vi "MCP3208 SPI Analog Input.vi"   [LabVIEW 2014]
doc: "This example shows how to read ADC value from MCP3208."
uses:
  QwaveSys_Interface/QwaveSys_Interface.lvlib
  PWS_ESP8266/PWS_ESP8266.lvlib
panel:
  # "Overview: Demonstrates how to read ADC data from MCP3208, Refer at this link: http://ww1.microchip.com/downloads/en/DeviceDoc/21298c.pdf\nRequirements: LabVIEW Full Development System,Arduino Compatible Compiler for LabVIEW,Programmable Wireless Stamp (PWS) Library.\nInstructions:\n1. Wire the MCP3208 IC to the Pmod SPI interface. refer below diagram.\n2. If this example has been loaded from the Arduino Compatible Compiler for LabVIEW, simply select Compile and Download.  Otherwise, open Tools>Arduino Compatible Compiler for LabVIEW in LabVIEW, then select File>Load VI, and select this VI and then Compile and Download.\n3. Open \"Serial Monitor\" by select \"Tools>Serial Monitor\" and select baud rate to 9600.\n4. Observe the data \"ADC 8 ch single end & 4 ch differential\" being print out on serial port monitor.\n\n#NOTE: \nThe MCP3208 chip is a very popular successive approximation 12-Bit ADC with SPI interface. The chip is programmable to provide four pseudo-differential input pairs or eight single-ended inputs and is capable of sample rates up to 100 Ksps. Custom designs or off the shelf modules utilizing the MCP3208 is a great option in case the user needs ADC channels with higher resolution than the 10-bit ADC that is included as part of the PWS.\nrefer: http://ww1.microchip.com/downloads/en/DeviceDoc/21298c.pdf"
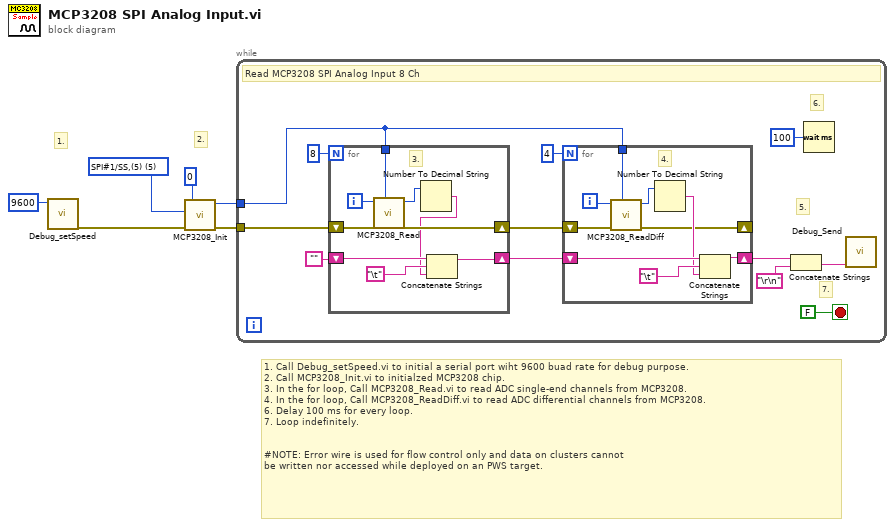
[diagram p0: block diagram]
diagram:
  w1 = u8 5 items=["SPI#1/SS,(5)"=5, "SPI#2/MOSI,(13)"=13, "SPI#3/MISO,(12)"=12, "SPI#4/SCLK,(14)"=14, "UART#1/CS,(15)"=15, "UART#2/TXD,(1)"=1, "UART#3/RXD,(3)"=3, "UART#4/LED,(16)"=16, "FPROM_Btn,(0)"=0, "SDCard_CS,(4)"=4, "I2C-SDA/TXD1,(2)"=2, "ADC0,(17)"=17] ("CS")
  # "2."
  # "1."
  # "1. Call Debug_setSpeed.vi to initial a serial port wiht 9600 buad rate for debug purpose.\n2. Call MCP3208_Init.vi to initialzed MCP3208 chip.\n3. In the for loop, Call MCP3208_Read.vi to read ADC single-end channels from MCP3208.\n4. In the for loop, Call MCP3208_ReadDiff.vi to read ADC differential channels from MCP3208.\n6. Delay 100 ms for every loop.\n7. Loop indefinitely.\n\n\n#NOTE: Error wire is used for flow control only and data on clusters cannot\nbe written nor accessed while deployed on an PWS target."
  n1 = call "Debug_setSpeed.vi"("Speed"=u32 9600) -> ("error out"=w3:errorcluster)  [unwired: 10 in]
  n2 = call "MCP3208_Init.vi"("error in"=w3, "CS"=w1, "Interface (0-4)"=u8 0) -> ("error out"=w4:errorcluster, "Instance"=w5:u8)  [unwired: 7 in]
  n3 = while {
    tunnel: w5 -> [w13]
    tunnel: w4 -> [w18]
    stop <- FALSE stop-if-true
    # "7."
    # "6."
    # "5."
    # "Read MCP3208 SPI Analog Input 8 Ch"
    n4 = for {
      N: 8 -> [_]
      shift-right: [w35] -> w8
      shift-left: w18 -> [w36]
      shift-right: [w33] -> w12
      shift-left: "" ("Empty String Constant") -> [w32]
      tunnel: w13 -> [w28]
      i -> [w34]
      # "3."
      n5 = call "MCP3208_Read.vi"("Instance"=w28, "error in (no error)"=w36, "Channel (0-7)"=w34) -> ("error out"=w35:errorcluster, "ADC"=w30:u16)  [unwired: 7 in]
      n6 = Number To Decimal String(number=w30) -> (decimal integer string=w29:string)  [unwired: 1 in]
      n7 = Concatenate Strings(w32, "\t" ("Tab Constant"), w29) -> (w33:string)
    }
    n8 = for {
      N: 4 -> [_]
      shift-right: [w22] -> _
      shift-left: w8 -> [w23]
      shift-right: [w27] -> w11
      shift-left: w12 -> [w26]
      tunnel: w13 -> [w20]
      i -> [w21]
      # "4."
      n9 = call "MCP3208_ReadDiff.vi"("Instance"=w20, "error in (no error)"=w23, "Channel (0-3)"=w21) -> ("error out"=w22:errorcluster, "Ch Diff ADC"=w19:i16)  [unwired: 7 in]
      n10 = Number To Decimal String(number=w19) -> (decimal integer string=w24:string)  [unwired: 1 in]
      n11 = Concatenate Strings(w26, "\t" ("Tab Constant"), w24) -> (w27:string)
    }
    n12 = Concatenate Strings(w11, "\r\n" ("End of Line Constant")) -> (w9:string)
    n13 = Wait (ms)(milliseconds to wait=u32 100) -> ()  [unwired: 1 out]
    n14 = call "Debug_Send.vi"("DATA"=w9) -> ()  [unwired: 11 in]
  }
